vi "Testing.vi"(8 "error in":errorcluster caption="error in (no error)") -> (0 "error out":errorcluster, 2 "Modules Out":string[][](array[string]), 3 "Chassis List Out":string[](array[string]))   [LabVIEW 2011]
uses:
  Controls/ModuleCluster.ctl
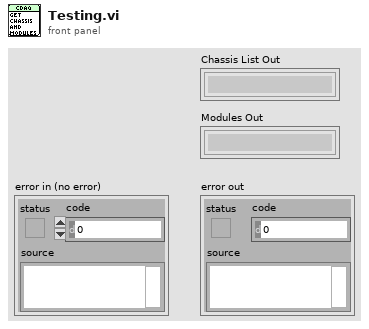
[diagram p1: front panel]
types:
  T1 = typedef "ModuleCluster.ctl" = cluster{"Device Ref":refnum<k20>, "ProdName":string, "ConnLink":string}
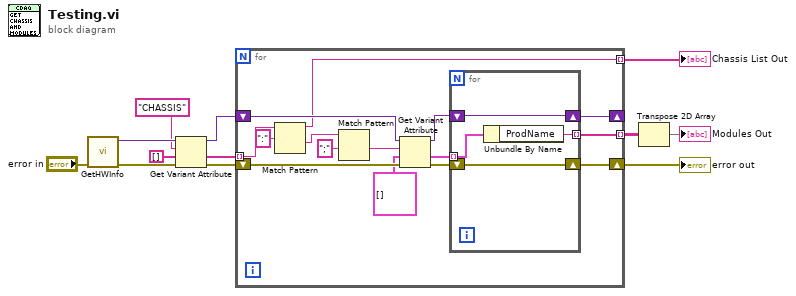
[diagram p0: block diagram]
diagram:
  n1 = call "GetHWInfo.vi"("error in"="error in") -> ("error out"=w12:errorcluster, "Refs Out"=w11:variant)  [unwired: 9 in]
  n2 = Get Variant Attribute(Variant=w11, name="CHASSIS", default value (empty Variant)=string[] [], error in=w12) -> (duplicate Variant=w6:variant, value=w7:string[], error out=w8:errorcluster)  [unwired: 1 out]
  n3 = for {
    shift-right: [w19] -> w3
    shift-left: w8 -> [w27]
    tunnel: w7 -> [w18] mode=indexing
    shift-right: [w21] -> _
    shift-left: w6 -> [w26]
    tunnel: [w20] -> w4 mode=indexing
    tunnel: [w17] -> w5 mode=indexing
    n4 = Match Pattern(string=w18, regular expression=":") -> (before substring=w17:string, after substring=w14:string)  [unwired: 1 in, 2 out]
    n5 = Match Pattern(string=w14, regular expression=";") -> (before substring=w13:string)  [unwired: 1 in, 3 out]
    n6 = Get Variant Attribute(Variant=w26, name=w13, default value (empty Variant)=T1[] [] ("appended array"), error in=w27) -> (duplicate Variant=w22:variant, value=w24:T1[], error out=w23:errorcluster)  [unwired: 1 out]
    n7 = for {
      tunnel: w24 -> [w30] mode=indexing
      shift-right: [w28] -> w19
      shift-left: w23 -> [w28]
      shift-right: [w31] -> w21
      shift-left: w22 -> [w31]
      tunnel: [w29] -> w20 mode=indexing
      n8 = Unbundle By Name(w30) -> ("ProdName"=w29:string)
    }
  }
  "Chassis List Out" <- w5
  "error out" <- w3
  n9 = Transpose 2D Array(2D array=w4) -> (transposed array=→"Modules Out":string[][])
